vi "Auto_Routine_LeaveCommunity.vi"(8 "error in (no error)":errorcluster) -> (0 "error out":errorcluster)   [LabVIEW 2023]
doc: "Leaves the community\n\ninput:\n--ErrorIn--\n\noutput:\n--ErrorOut--"
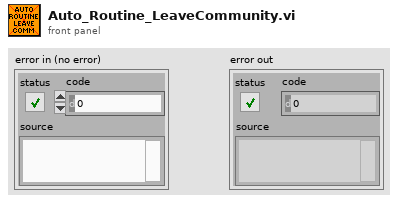
[diagram p1: front panel]
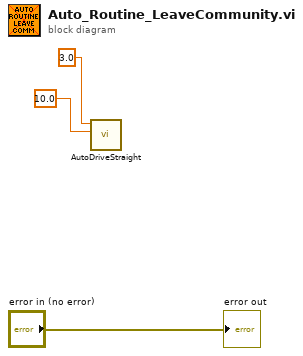
[diagram p0: block diagram]
diagram:
  n1 = call "AutoDriveStraight.vi"("MaxSpeed (ft/s)"=10.0, "Dist (ft)"=3.0) -> ()  [unwired: 9 in, 1 out]
  "error out" <- "error in (no error)"
